vi "COMMAND_GetCurrentPosition.vi"(8 "error in (no error)":errorcluster, 11 "MH100301DMC in":refnum<class "StageMH100301DMC.lvclass">) -> (0 "error out":errorcluster, 2 "current position":refnum<class "SpaceVector.lvclass">, 3 "MH100301DMC out":refnum<class "StageMH100301DMC.lvclass">)   [LabVIEW 2010, in "StageMH100301DMC.lvclass"]
uses:
  StageMH100301DMC.lvclass
  common/classes/SpaceVector/SpaceVector/SpaceVector.lvclass
  StageMH100301DMC.lvclass/StageMH100301DMC.ctl
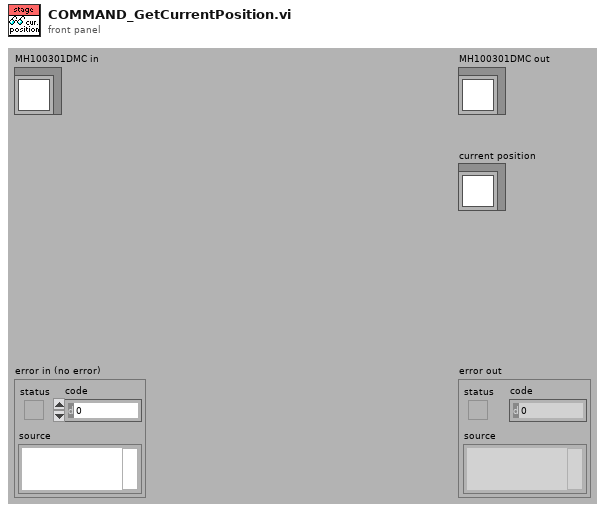
[diagram p1: front panel]
types:
  T1 = cluster{"[0]":dbl[unit], "[1]":dbl[unit], "[2]":dbl[unit]}
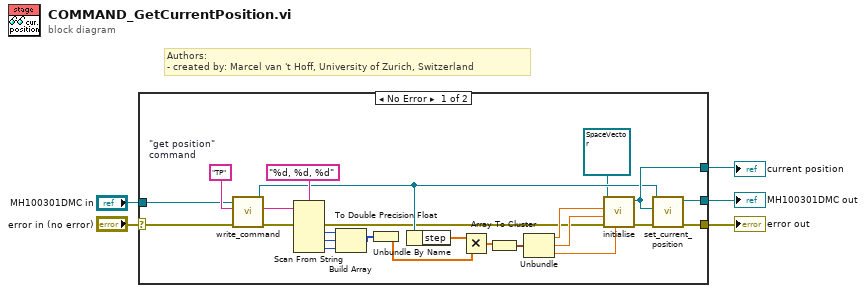
[diagram p0: block diagram]
diagram:
  # "Authors: \n- created by: Marcel van 't Hoff, University of Zurich, Switzerland"
  n1 = case shown="No Error" "error in (no error)" {
    selector: "error in (no error)" -> [w7 w31]
    tunnel: [w28 w31] -> w4
    tunnel: [w26 w30] -> w2
    tunnel: "MH100301DMC in" -> [w27 w30]
    tunnel: [w25 _] -> w1
    frame No Error {
      w29 = "TP"  # "get position"  command
      n2 = call-dynamic "write_command.vi"("error in (no error)"=w7, "command (without terminating \"\\n\")"=w29, "MH100301DMC in"=w27) -> ("error out"=w16:errorcluster, "response out"=w17:string, "MH100301DMC out"=w12:refnum<class "StageMH100301DMC.lvclass">)  [unwired: 6 out]
      n3 = Scan From String(format string="%d, %d, %d", input string=w17, error in=w16) -> (error out=w9:errorcluster, output 1=w15:i32, output 2=w14:i32, output 3=w13:i32)  [unwired: 1 in, 5 out]
      n4 = Build Array(w15, w14, w13) -> (w24:i32[])
      n5 = To Double Precision Float(number=w24) -> (double precision float=w11:dbl[])
      n6 = Unbundle By Name(w12) -> ("step"=w10:dbl[unit][])
      n7 = Multiply(x=w10, y=w11) -> (x*y=w8:dbl[unit][])
      n8 = Array To Cluster(array=w8) -> (cluster=w22:T1)
      n9 = Unbundle(w22) -> ("[0]"=w21:dbl[unit], "[1]"=w20:dbl[unit], "[2]"=w19:dbl[unit])
      n10 = call "initialise.vi"("z"=w19, "error in (no error)"=w9, "y"=w20, "x"=w21, "SpaceVector in"=refnum<class "SpaceVector.lvclass"> refnum) -> ("error out"=w23:errorcluster, "SpaceVector out"=w25:refnum<class "SpaceVector.lvclass">)  [unwired: 5 out]
      n11 = call-dynamic "set_current_position.vi"("error in (no error)"=w23, "current position"=w25, "DL090409StageScaffold.lvclass in"=w12) -> ("error out"=w28:errorcluster, "DL090409StageScaffold.lvclass out"=w26:refnum<class "StageMH100301DMC.lvclass">)  [unwired: 7 out]
    }
    frame Error {
    }
  }
  "error out" <- w4
  "MH100301DMC out" <- w2
  "current position" <- w1
